vi "Confirm Command.vi"(11 "Extracted Data Set":u8[](array[numeric])) -> (3 "Full command received":bool)   [LabVIEW 2011]
doc: "This VI checks the fletcher checksum of the recived data vs the checksum sent with the data.\n\nReturns if the checksums are correct."
panel:
  out "Checksum LSB":u8
  out "Checksum MSB":u8
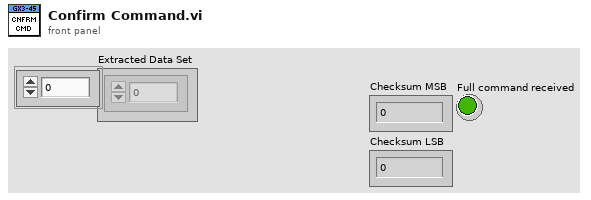
[diagram p1: front panel]
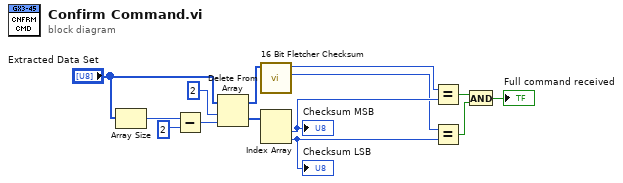
[diagram p0: block diagram]
diagram:
  n1 = Array Size(array="Extracted Data Set") -> (size(s)=w14:i32)
  n2 = Subtract(x=w14, y=2) -> (x-y=w11:i32)
  n3 = Delete From Array(array="Extracted Data Set", length=2, index=w11) -> (deleted portion=w9:u8[], array with subset deleted=w8:u8[])
  n4 = call "16 Bit Fletcher Checksum.vi"("Input Array"=w8) -> ("B (LSB)"=w5:u8, "A (MSB)"=w6:u8)  [unwired: 8 in, 1 out]
  n5 = Index Array(array=w9) -> (element #1=w7:u8, element #2=w4:u8)  [unwired: 2 in]
  "Checksum MSB" <- w7
  "Checksum LSB" <- w4
  n6 = Equal?(x=w6, y=w7) -> (x = y?=w3:bool)
  n7 = Equal?(x=w5, y=w4) -> (x = y?=w2:bool)
  n8 = And(x=w3, y=w2) -> (x .and. y?=→"Full command received":bool)
